vi "fn Create Demo Group.vi"(8 "error in (no error)":errorcluster) -> (0 "error out":errorcluster, 3 "function return":i32)   [LabVIEW 2018, in "LV_OPC.lvlib"]
doc: "LVOPC_API int fnCreateDemoGroup();"
uses:
  LV_OPC.lvlib
  LVOPC64.dll
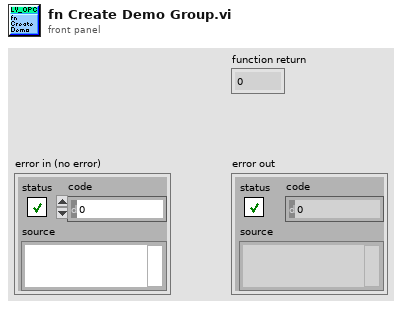
[diagram p1: front panel]
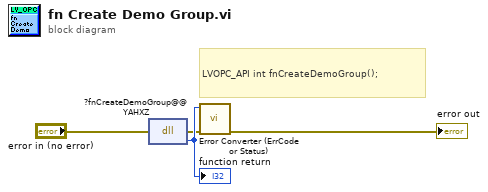
[diagram p0: block diagram]
diagram:
  # "LVOPC_API int fnCreateDemoGroup();"
  n1 = dll-call lib="C:/Users/Andrey/Desktop/LV_OPC-Client-x64/LV_OPC_Test/OPC.DLL/LVOPC64.*" fn="?fnCreateDemoGroup@@YAHXZ"(error in="error in (no error)") -> (error out=w2:errorcluster, "return type"=w4:i32)  [unwired: 2 in, 1 out]
  "function return" <- w4
  n2 = call "Error Converter (ErrCode or Status).vi"("error in (no error)"=w2, "error code"=w4) -> ("error out"=→"error out":errorcluster)  [unwired: 9 in]
